vi "Load Config.vi"(6 "Constants":refnum<class "Sequence Constants.lvclass">, 8 "error in (no error)":refnum<class "MultiErrors.lvclass">, 10 "Config Element":refnum<class "Config Element.lvclass">, 11 "HighLimit Condition Config in":refnum<class "HighLimit Condition Config.lvclass">) -> (0 "error out":refnum<class "MultiErrors.lvclass">, 3 "HighLimit Condition Config out":refnum<class "HighLimit Condition Config.lvclass">)   [LabVIEW 2020, in "VolatusSeqConfig.lvlib" / "HighLimit Condition Config.lvclass"]
uses:
  HighLimit Condition Config.lvclass
  VolatusErrorUtilities/MultiErrors/MultiErrors.lvclass
  lv-cdm/CDM-Config/Config Element/Config Element.lvclass
  HighLimit Condition Config.lvclass/HighLimit Condition Config.ctl
  Sequence Constants/Sequence Constants.lvclass
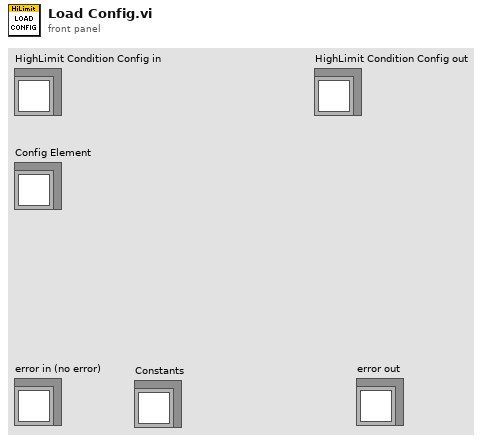
[diagram p1: front panel]
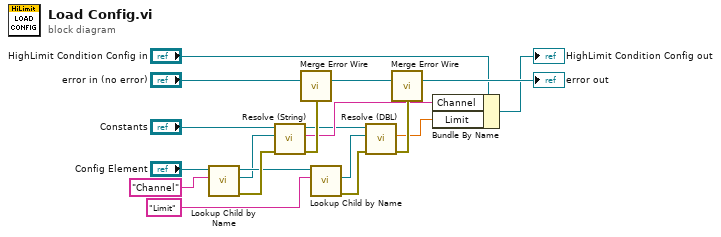
[diagram p0: block diagram]
diagram:
  n1 = call "Lookup Child by Name.vi"("Name"="Channel", "Config Element in"="Config Element") -> ("error out"=w19:errorcluster, "Child"=w9:refnum<class "Config Element.lvclass">, "Config Element out"=w11:refnum<class "Config Element.lvclass">)  [unwired: 6 in, 1 out]
  n2 = call "Resolve (String).vi"("error in (no error)"=w19, "Element"=w9, "Sequence Constants in"="Constants") -> ("error out"=w16:errorcluster, "String Value"=w7:string, "Sequence Constants out"=w1:refnum<class "Sequence Constants.lvclass">)  [unwired: 6 in]
  n3 = call "Merge Error Wire.vi"("error in (no error)"=w16, "MultiErrors in"="error in (no error)") -> ("MultiErrors out"=w3:refnum<class "MultiErrors.lvclass">)  [unwired: 13 in]
  n4 = call "Lookup Child by Name.vi"("Name"="Limit", "Config Element in"=w11) -> ("error out"=w4:errorcluster, "Child"=w6:refnum<class "Config Element.lvclass">)  [unwired: 6 in, 2 out]
  n5 = call "Resolve (DBL).vi"("error in (no error)"=w4, "Element"=w6, "Sequence Constants in"=w1) -> ("error out"=w17:errorcluster, "DBL Value"=w5:dbl)  [unwired: 6 in, 1 out]
  n6 = call "Merge Error Wire.vi"("error in (no error)"=w17, "MultiErrors in"=w3) -> ("MultiErrors out"=→"error out":refnum<class "MultiErrors.lvclass">)  [unwired: 13 in]
  n7 = Bundle By Name(cluster="HighLimit Condition Config in", "Channel"=w7, "Limit"=w5) -> (→"HighLimit Condition Config out":refnum<class "HighLimit Condition Config.lvclass">)
